vi "dbInsert_subVI.vi"(8 "Enum":T1, 9 "Array":sgl[](array[numeric]), 10 "reference":refnum<k24>) -> ()   [LabVIEW 2015]
uses:
  DBEnum.ctl
  C:/Users/Arkadiusz/SkyDrive/Dokumenty/NordicSemiconductor/LabVIEW/UART_Accelero/uart data_akcelerometr/NordicDatabaseDLL.dll
  NordicDatabaseDLL.dll
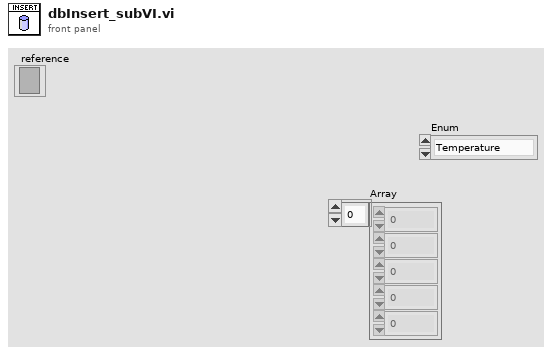
[diagram p1: front panel]
types:
  T1 = typedef "DBEnum.ctl" = enum16{"Temperature", "HeartRate", "XAccelero", "YAccelero", "ZAccelero"}
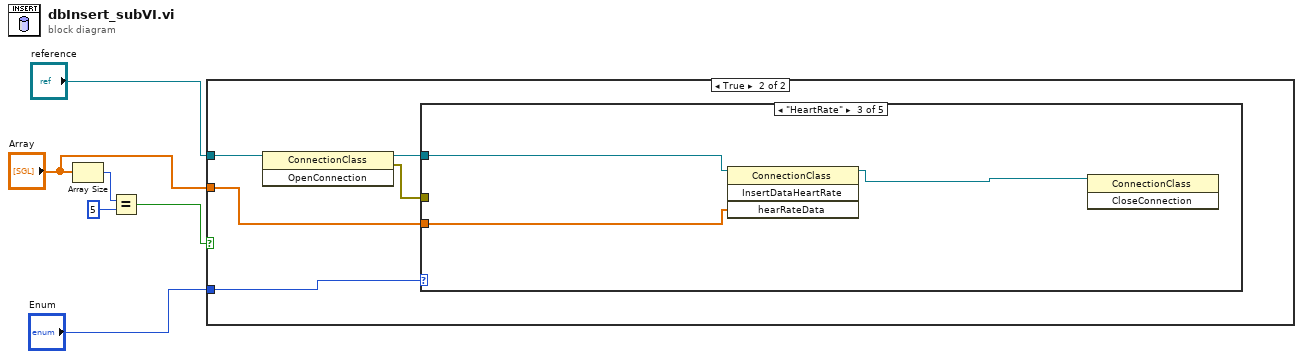
[diagram p0: block diagram]
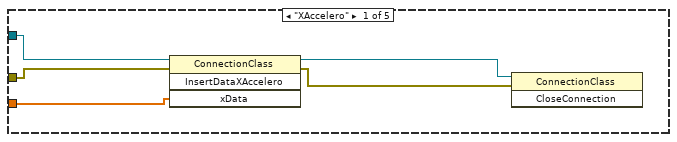
[diagram p3: hidden frame]
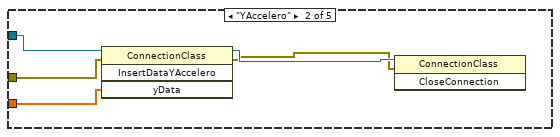
[diagram p4: hidden frame]
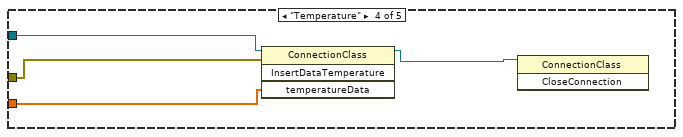
[diagram p5: hidden frame]
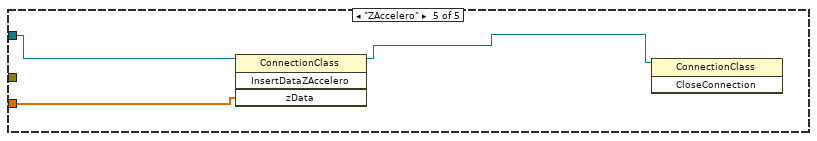
[diagram p6: hidden frame]
diagram:
  n1 = Array Size(array="Array") -> (size(s)=w5:i32)
  n2 = Equal?(x=w5, y=5) -> (x = y?=w3:bool)
  n3 = case shown="True" w3 {
    tunnel: "Enum" -> [_ w11]
    tunnel: "Array" -> [_ w10]
    tunnel: "reference" -> [_ w7]
    frame False {
    }
    frame True {
      n4 = invoke class="ConnectionClass" method="OpenConnection"(reference=w7) -> (reference out=w9:refnum<k24>, error out=w8:errorcluster)  [unwired: 2 in, 1 out]
      n5 = case shown="\"HeartRate\"" w11 {
        tunnel: w10 -> [w15 w21 w24 w28 w31]
        tunnel: w9 -> [w16 w19 w22 w26 w29]
        tunnel: w8 -> [w14 w18 _ w25 _]
        frame "XAccelero" {
          n6 = invoke class="ConnectionClass" method="InsertDataXAccelero"(reference=w16, error in=w14, "xData"=w15) -> (reference out=w13:refnum<k24>, error out=w12:errorcluster)  [unwired: 1 in, 2 out]
          n7 = invoke class="ConnectionClass" method="CloseConnection"(reference=w13, error in=w12) -> ()  [unwired: 1 in, 3 out]
        }
        frame "YAccelero" {
          n8 = invoke class="ConnectionClass" method="InsertDataYAccelero"(reference=w19, error in=w18, "yData"=w21) -> (reference out=w20:refnum<k24>, error out=w17:errorcluster)  [unwired: 1 in, 2 out]
          n9 = invoke class="ConnectionClass" method="CloseConnection"(reference=w20, error in=w17) -> ()  [unwired: 1 in, 3 out]
        }
        frame "HeartRate" {
          n10 = invoke class="ConnectionClass" method="InsertDataHeartRate"(reference=w22, "hearRateData"=w24) -> (reference out=w23:refnum<k24>)  [unwired: 2 in, 3 out]
          n11 = invoke class="ConnectionClass" method="CloseConnection"(reference=w23) -> ()  [unwired: 2 in, 3 out]
        }
        frame "Temperature" {
          n12 = invoke class="ConnectionClass" method="InsertDataTemperature"(reference=w26, error in=w25, "temperatureData"=w28) -> (reference out=w27:refnum<k24>)  [unwired: 1 in, 3 out]
          n13 = invoke class="ConnectionClass" method="CloseConnection"(reference=w27) -> ()  [unwired: 2 in, 3 out]
        }
        frame "ZAccelero" {
          n14 = invoke class="ConnectionClass" method="InsertDataZAccelero"(reference=w29, "zData"=w31) -> (reference out=w30:refnum<k24>)  [unwired: 2 in, 3 out]
          n15 = invoke class="ConnectionClass" method="CloseConnection"(reference=w30) -> ()  [unwired: 2 in, 3 out]
        }
      }
    }
  }
